vi "Actor Core.vi"(8 "error in":errorcluster, 11 "ReceiverState in":refnum<class "Connect Command.lvclass">) -> (0 "error out":errorcluster, 3 "Actor out":refnum<class "Actor.lvclass">)   [LabVIEW 2013, in "Receiver.lvlib" / "Receive Commands Using State Actors.lvlib" / "Connect Command.lvlib" / "Connect Command.lvclass"]
doc: "(<B>Filename</B>: Actor Framework.lvlib:Actor.lvclass:Actor Core.vi)\n\nReceives messages to the actor, reacts to them, and initiates any error handling that may shut the actor down.\n\nDescendant classes may override this VI to append parallel tasks for the actor to complete while it handles messages. Overrides use the Call Parent Method node."
uses:
  Connect Command.lvclass
  <vilib>/ActorFramework/Actor/Actor.lvclass
  Receiver Commands/Receiver Command.lvclass
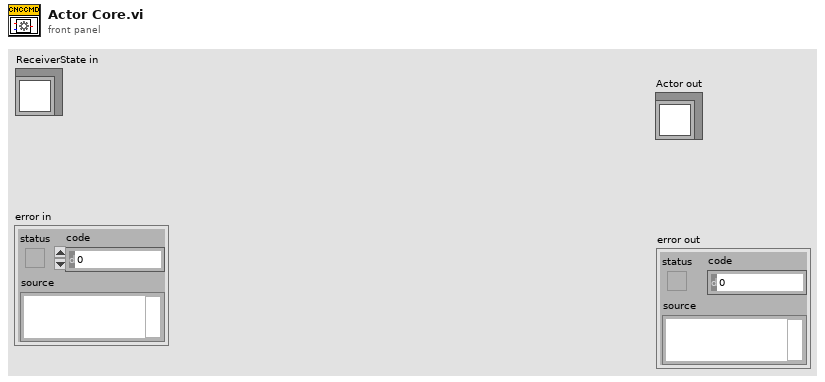
[diagram p1: front panel]
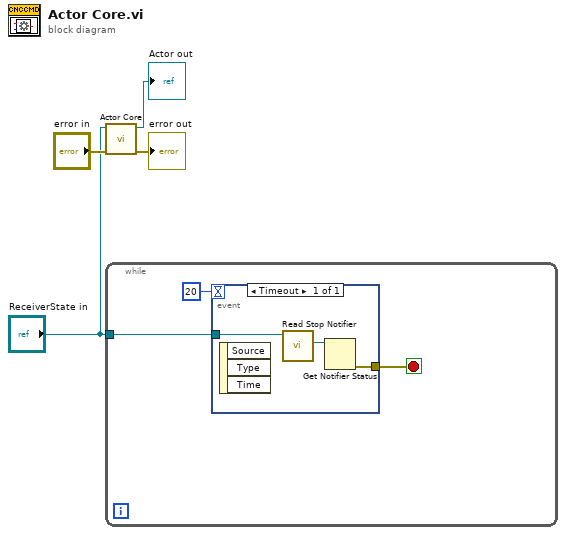
[diagram p0: block diagram]
diagram:
  n1 = call-parent "Actor Core.vi"("error in"="error in", "State in"="ReceiverState in") -> ("error out"=→"error out":errorcluster, "Actor out"=→"Actor out":refnum<class "Actor.lvclass">)  [unwired: 8 in]
  n2 = while {
    tunnel: "ReceiverState in" -> [w6]
    stop <- w5 stop-if-true
    n3 = event shown="[0] Timeout" {
      selector: _ -> [_]
      dyn-events: _ -> [_]
      timeout: 20 -> [_]
      tunnel: w6 -> [w9]
      tunnel: [w10] -> w5
      event Timeout {
        n4 = event-data() -> ()  [unwired: 1 in, 3 out]
        n5 = call-dynamic "Read Stop Notifier.vi"("Command in"=w9) -> ("Stop Notifier"=w8:refnum<notifier>)  [unwired: 8 in, 2 out]
        n6 = Get Notifier Status(notifier=w8) -> (error out=w10:errorcluster)  [unwired: 1 in, 4 out]
      }
    }
  }
